vi "PicoLogDriver.vi"(1 "stop":bool) -> ()   [LabVIEW 2016]
uses:
  <vilib>/Platform/TimedLoop/XDataNode/timing_clust.ctl
  <vilib>/Platform/TimedLoop/XDataNode/nitl_modes.ctl
  <vilib>/Platform/TimedLoop/XDataNode/wakeup.ctl
  <vilib>/Utility/NIReport.llb/image depth.ctl
  Instance           1 30Saved   pl1000StreamingExample .vi
  <vilib>/Utility/NIReport.llb/Append Report Text (str wrap).vi
  <vilib>/printing/OpenHTMLReport.llb/Open HTML Report in Browser (Refnum).vi
  <vilib>/platform/TimedLoop/XDataNode/XDataNode.xnode
  <vilib>/Utility/NIReport.llb/NI_report.lvclass
  pl1000.dll
  <vilib>/Platform/TimedLoop/XDataNode/XDNodeRunTimeDep.lvlib
  <vilib>/Utility/NIReport.llb/NI_ReportGenerationCore.lvlib
panel:
  in  "Tab Control":enum32{"Real Time", "Over time"}(tab)
  out "Waveform Chart":dbl[][](graph)
  out "Vin":dbl format="%#.2f"
  out "Elapsed Time":string caption="Elapsed Time Text"
  out "Time variation Graph":waveform(dbl)[](graph)
  out "error out 2":errorcluster
  out "Boolean":bool
  out "Path":path
  in  "Period (microseconds)":u16=100 min=100 max=1800
  out "Triggered":bool
  out "No. of channels":i32
  in  "D3":bool=TRUE
  in  "D2":bool=TRUE
  in  "D1":bool=TRUE
  in  "D0":bool=TRUE
  in  "Enable auto trigger":bool
  in  "Trigger Enable":bool
  in  "Hysteresis (mV)":u32
  in  "Threshold (mV)":u32=1000
  in  "Trigger direction":u16(ring) items=["Rising", "Falling"]
  in  "Trigger channel":u16=1 min=1 max=16 step=1
  in  "Auto trigger time (ms)":u16=1000
  out "Sampling rate (S/s)":dbl
  in  "Channels Enabled (e.g 1,2,3,4) * use comma*":string="1,2,3,4,5"
  in  "Desired sample rate (S/s)":u32=100 max=100000
  # "Trigger Settings"
  # "CH5 - Vin"
  # "CH4 - temperature sensor"
  # "Current Values in mV"
  # "CH1"
  # "CH2"
  # "CH3"
  # "Temperature"
  # "@Vlad-Eusebiu Baciu"
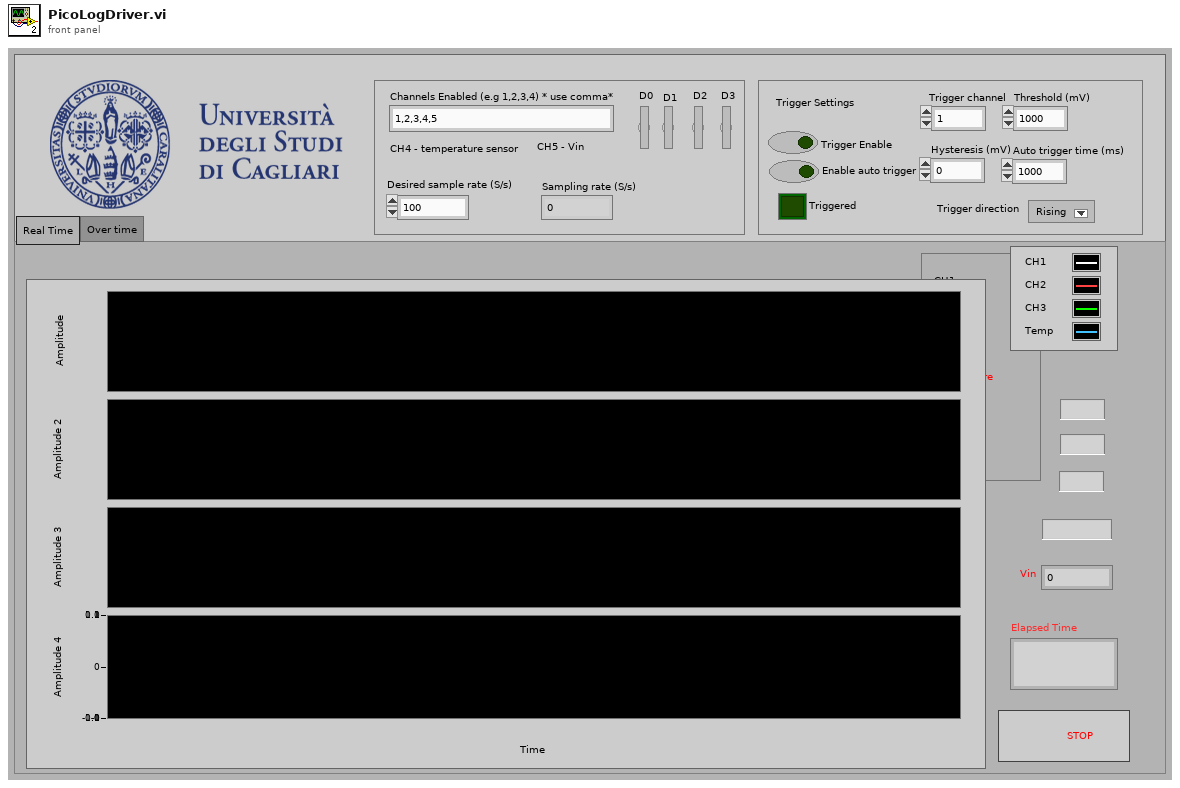
[diagram p1: front panel]
types:
  T1 = enum16{"open", "open or create", "create or replace", "create", "open (read-only)"}
  T2 = typedef "XDNodeRunTimeDep.lvlib/timing_clust.ctl" = cluster{"Expected End [f-1]":u64, "Actual End [f-1]":u64, "Finished Late? [f-1]":bool, "Expected End [i-1]":u64, "Actual End [i-1]":u64, "Finished Late? [i-1]":bool, "Expected Start [i]":u64, "Actual Start [i]":u64, "Expected Start [f]":u64, "Actual Start [f]":u64, "Source Name":string, "Structure Name":string, "Period":i64, "Deadline":i64, "Offset":i64, "Start":i64, "Priority":i32, "Timeout":i32, "Mode":T3, "Wakeup Reason":T4, "Error":errorcluster, "Source Type":string, "Secondary Source Type":string, "Global End Time":u64, "Global Start Time":u64, "Frame Duration":u64, "Iteration Duration":u64, "Assigned CPU":i32, "I/O Scan Engine Mode":u32}
  T3 = typedef "XDNodeRunTimeDep.lvlib/nitl_modes.ctl" = enum32{"No Change", "Process missed periods, maintain original phase", "Discard missed periods, maintain original phase", "Process missed periods, ignore original phase", "Discard missed periods, ignore original phase"}
  T4 = typedef "XDNodeRunTimeDep.lvlib/wakeup.ctl" = enum32{"Normal", "Aborted", "Asynchronous wakeup", "Timing source error", "Timed loop error", "Timeout"}
  T5 = enum8{"Enabled", "Disabled", "Disabled and Grayed Out"}
  T6 = enum16{"Standard Report", "HTML", "Word", "Excel"}
  T7 = typedef "NI_ReportGenerationCore.lvlib/image depth.ctl" = u16
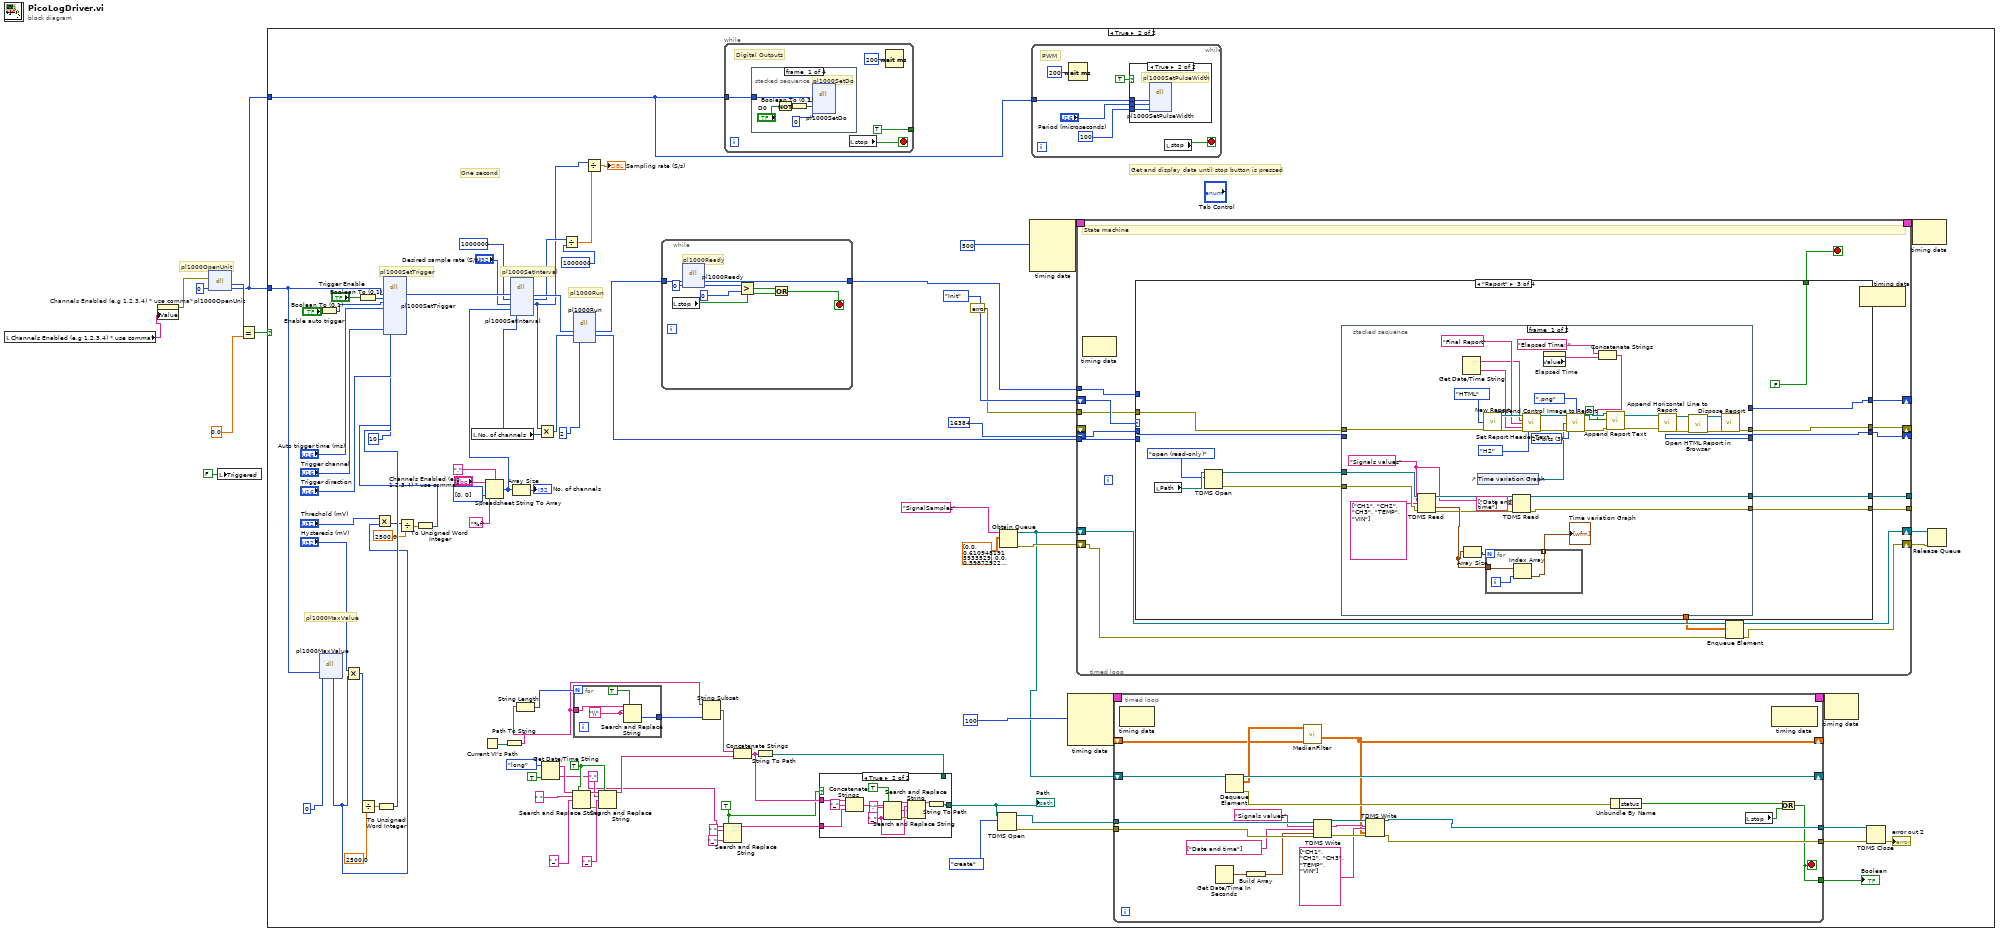
[diagram p0: block diagram]
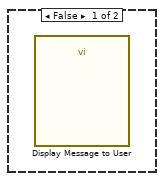
[diagram p2: hidden frame]
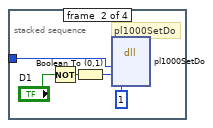
[diagram p5: hidden frame]
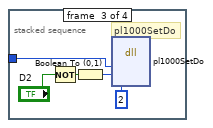
[diagram p6: hidden frame]
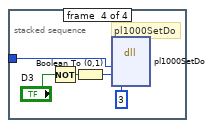
[diagram p7: hidden frame]
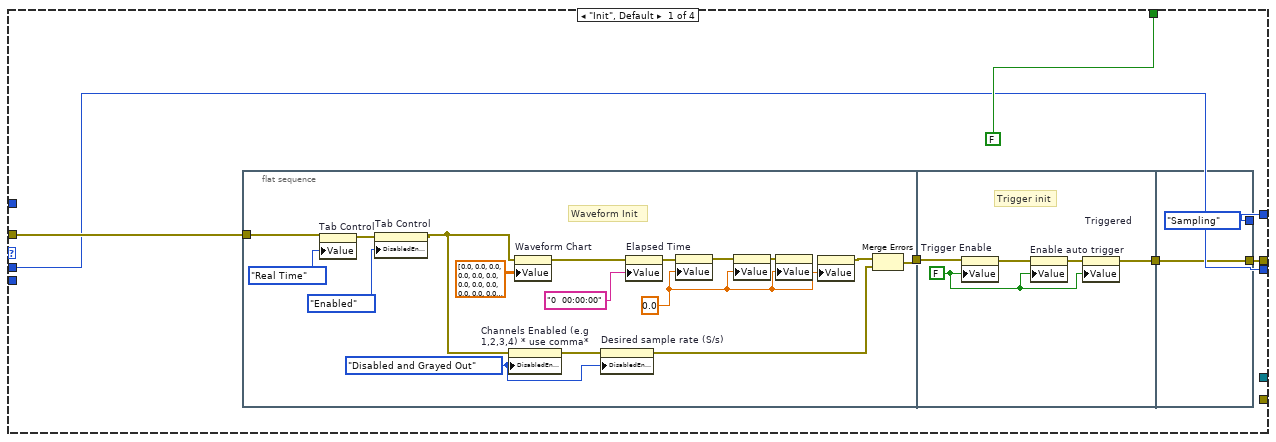
[diagram p8: hidden frame]
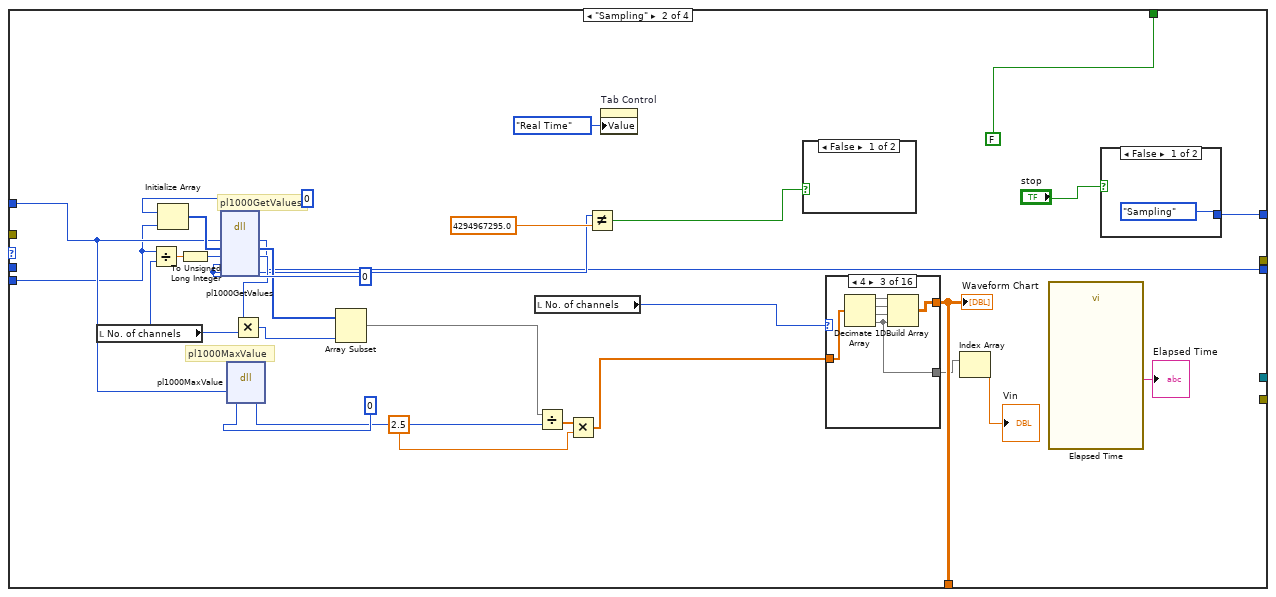
[diagram p9: hidden frame]
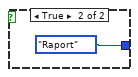
[diagram p10: hidden frame]
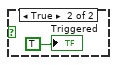
[diagram p11: hidden frame]
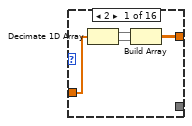
[diagram p12: hidden frame]
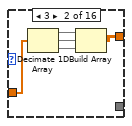
[diagram p13: hidden frame]
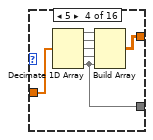
[diagram p14: hidden frame]
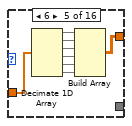
[diagram p15: hidden frame]
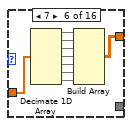
[diagram p16: hidden frame]
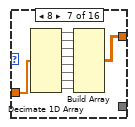
[diagram p17: hidden frame]
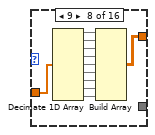
[diagram p18: hidden frame]
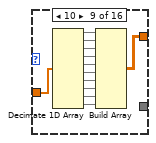
[diagram p19: hidden frame]
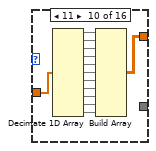
[diagram p20: hidden frame]
diagram:
  # "pl1000OpenUnit"
  n1 = local read "Channels Enabled (e.g 1,2,3,4) * use comma*"() -> (w1:string)
  n2 = property on="Channels Enabled (e.g 1,2,3,4) * use comma*" class="Str"("Value"=w1) -> (error out=w2:errorcluster)  [unwired: 2 in, 1 out]
  n3 = dll-call lib="E:/Erasmus practica/pl1000.dll" fn="pl1000OpenUnit"(error in=w2, "handle"=i16 0) -> ("status"=w5:u32, "handle"=w4:i16)  [unwired: 2 in, 2 out]
  n4 = local write "Triggered"(FALSE ("Boolean")) -> ()
  n5 = Equal?(x=w5, y=0.0) -> (x = y?=w7:bool)
  n6 = case shown="True" w7 {
    tunnel: w4 -> [_ w77]
    tunnel: w4 -> [_ w49]
    frame False {
      n7 = call "Display Message to User"() -> ()  [unwired: 10 in, 2 out]
    }
    frame True {
      w13 = TRUE ("replace all? (F)")
      w31 = TRUE ("replace all? (F)")
      # "Get and display data until stop button is pressed"
      # "One second"
      # "pl1000MaxValue"
      # "pl1000SetTrigger"
      # "pl1000Run"
      # "pl1000SetInterval"
      n8 = dll-call lib="E:/Erasmus practica/pl1000.dll" fn="pl1000MaxValue"("handle"=w77, "maxValue"=u16 0) -> ("maxValue"=w67:u16)  [unwired: 5 in, 2 out]
      n9 = Boolean To (0,1)(Boolean="Enable auto trigger") -> (0, 1=w57:i16)
      n10 = Multiply(x="Hysteresis (mV)", y=w67) -> (x*y=w79:u32)
      n11 = Boolean To (0,1)(Boolean="Trigger Enable") -> (0, 1=w65:i16)
      n12 = Divide(x=w79, y=2500.0) -> (x/y=w74:dbl)
      n13 = Multiply(x="Threshold (mV)", y=w67) -> (x*y=w70:u32)
      n14 = To Unsigned Word Integer(number=w74) -> (unsigned 16bit integer=w75:u16)
      n15 = Divide(x=w70, y=2500.0) -> (x/y=w71:dbl)
      n16 = To Unsigned Word Integer(number=w71) -> (unsigned 16bit integer=w68:u16)
      n17 = dll-call lib="E:/Erasmus practica/pl1000.dll" fn="pl1000SetTrigger"("handle"=w77, "enabled"=w65, "auto_trigger"=w57, "auto_ms"="Auto trigger time (ms)", "channel"="Trigger channel", "dir"="Trigger direction", "threshold"=w68, "hysteresis"=w75, "delay"=u16 10) -> ("handle"=w97:i16)  [unwired: 12 in, 2 out]
      n18 = local read "No. of channels"() -> (w62:i32)
      n19 = Current VI's Path() -> (path=w39:path)
      n20 = Spreadsheet String To Array(delimiter (Tab)=",", format string="%f", spreadsheet string="Channels Enabled (e.g 1,2,3,4) * use comma*", array type (2D Dbl)=u32[] [0, 0]) -> (array=w89:u32[])
      n21 = Path To String(path=w39) -> (string=w28:string)
      n22 = dll-call lib="E:/Erasmus practica/pl1000.dll" fn="pl1000SetInterval"("handle"=w97, "us_for_block"=u32 1000000, "ideal_no_of_samples"="Desired sample rate (S/s)", "channels"=w89, "no_of_channels"=w62) -> ("handle"=w94:i16, "us_for_block"=w84:u32, "ideal_no_of_samples"=w61:u32)  [unwired: 6 in, 2 out]
      n23 = Array Size(array=w89) -> (size(s)=→"No. of channels":i32)
      n24 = String Length(string=w28) -> (length=w30:i32)
      n25 = Multiply(x=w61, y=w62) -> (x*y=w60:u32)
      n26 = Get Date/Time String(date format (0)=enum16{"short", "long", "abbreviated"}."long", want seconds? (F)=TRUE) -> (date string=w37:string, time string=w23:string)  [unwired: 1 in]
      n27 = Divide(x=w84, y=u32 1000000) -> (x/y=w83:dbl)
      n28 = Search and Replace String(replace all?=w31, input string=w37, search string=" ", replace string="_" ("replace string (\"\")")) -> (result string=w35:string, error out=w25:errorcluster)  [unwired: 4 in, 2 out]
      n29 = dll-call lib="E:/Erasmus practica/pl1000.dll" fn="pl1000Run"("handle"=w94, "no_of_values"=w60, "method"=2) -> ("handle"=w95:i16, "no_of_values"=w86:u32)  [unwired: 5 in, 2 out]
      n30 = for {
        N: w30 -> [_]
        tunnel: w28 -> [w113]
        tunnel: [w112] -> w29
        w110 = "\\" ("regular expression")
        n31 = Search and Replace String(replace all?=TRUE ("replace all? (F)"), input string=w113, search string=w110, replace string=w110) -> (offset past replacement=w112:i32)  [unwired: 4 in, 3 out]
      }
      n32 = Divide(x=w61, y=w83) -> (x/y=→"Sampling rate (S/s)":dbl)
      n33 = Search and Replace String(replace all?=w31, input string=w35, search string=",", replace string="_" ("replace string (\"\")"), error in=w25) -> (result string=w27:string)  [unwired: 3 in, 3 out]
      n34 = while {
        tunnel: w95 -> [w512]
        tunnel: [w511] -> w93
        stop <- w507 stop-if-true
        # "pl1000Ready"
        n35 = local read "stop"() -> (w506:bool)
        n36 = dll-call lib="E:/Erasmus practica/pl1000.dll" fn="pl1000Ready"("handle"=w512, "ready"=i16 0) -> ("handle"=w511:i16, "ready"=w508:i16)  [unwired: 4 in, 2 out]
        n37 = Greater?(x=w508, y=i16 0) -> (0:w509:bool)
        n38 = Or(x=w509, y=w506) -> (x .or. y?=w507:bool)
      }
      n39 = String Subset(string=w28, length (rest)=w29) -> (substring=w26:string)  [unwired: 1 in]
      n40 = Search and Replace String(replace all?=w13, input string=w23, search string=" ", replace string="_" ("replace string (\"\")")) -> (result string=w20:string)  [unwired: 4 in, 3 out]
      n41 = while {
        tunnel: [TRUE] -> _
        tunnel: w49 -> [w150]
        stop <- w153 stop-if-true
        # "Digital Outputs"
        n42 = stacked-sequence {
          tunnel: w150 -> [w154 w159 w164 w169]
          frame #0 {
            # "pl1000SetDo"
            n43 = Not(x="D0") -> (.not. x?=w155:bool)
            n44 = Boolean To (0,1)(Boolean=w155) -> (0, 1=w157:i16)
            n45 = dll-call lib="E:/Erasmus practica/pl1000.dll" fn="pl1000SetDo"("handle"=w154, "do_value"=w157, "doNo"=i16 0) -> ()  [unwired: 7 in, 2 out]
          }
          frame #1 {
            # "pl1000SetDo"
            n46 = Not(x="D1") -> (.not. x?=w160:bool)
            n47 = Boolean To (0,1)(Boolean=w160) -> (0, 1=w162:i16)
            n48 = dll-call lib="E:/Erasmus practica/pl1000.dll" fn="pl1000SetDo"("handle"=w159, "do_value"=w162, "doNo"=i16 1) -> ()  [unwired: 7 in, 2 out]
          }
          frame #2 {
            # "pl1000SetDo"
            n49 = Not(x="D2") -> (.not. x?=w165:bool)
            n50 = Boolean To (0,1)(Boolean=w165) -> (0, 1=w167:i16)
            n51 = dll-call lib="E:/Erasmus practica/pl1000.dll" fn="pl1000SetDo"("handle"=w164, "do_value"=w167, "doNo"=i16 2) -> ()  [unwired: 7 in, 2 out]
          }
          frame #3 {
            # "pl1000SetDo"
            n52 = Not(x="D3") -> (.not. x?=w170:bool)
            n53 = Boolean To (0,1)(Boolean=w170) -> (0, 1=w172:i16)
            n54 = dll-call lib="E:/Erasmus practica/pl1000.dll" fn="pl1000SetDo"("handle"=w169, "do_value"=w172, "doNo"=i16 3) -> ()  [unwired: 7 in, 2 out]
          }
        }
        n55 = local read "stop"() -> (w153:bool)
        n56 = Wait (ms)(milliseconds to wait=u32 200) -> ()  [unwired: 1 out]
      }
      n57 = Concatenate Strings(w26, w27) -> (w24:string)
      n58 = String To Path(string=w24) -> (path=w12:path)
      n59 = case shown="True" w13 {
        tunnel: w24 -> [_ w109]
        tunnel: w20 -> [_ w107]
        tunnel: [w98 w106] -> w14
        tunnel: w12 -> [w98 _]
        frame False {
        }
        frame True {
          w101 = "_" ("replace string (\"\")")
          w100 = ":" ("search string")
          n60 = Concatenate Strings(w109, "_" ("string"), w107) -> (w105:string)
          n61 = Search and Replace String(replace all?=TRUE ("replace all? (F)"), input string=w105, search string=w100, replace string=w101) -> (result string=w102:string, error out=w103:errorcluster)  [unwired: 4 in, 2 out]
          n62 = Search and Replace String(input string=w102, search string=w101, replace string=w100, error in=w103) -> (result string=w99:string)  [unwired: 4 in, 3 out]
          n63 = String To Path(string=w99) -> (path=w106:path)
        }
      }
      "Path" <- w14
      n64 = TDMS Open(10:T1."create" ("operation (0:open)"), 11:w14) -> (0:w16:errorcluster, 3:w17:refnum<k34>)  [unwired: 5 in]
      n65 = Obtain Queue(name (unnamed)="SignalSamples", element data type=dbl[][] [[0.0, 0.6109481915933529, 0.0, 0.5987292277614858, 0.0, 0.6036168132942327, 0.0, 0.6085043988269795, 0.0, 0.6085043988269795, 0.0, 0.6133919843597263, 0.0, 0.6207233626588465, 0.0, 0.4056695992179863, 0.0, 0.4032258064516129, 0.0, 0.4032258064516129, 0.0, 0.4105571847507331, 0.0, 0.4105571847507331, 0.0, 0.4130009775171065, 0.0, 0.4130009775171065, 0.0, 0.760019550342131, 0.0, 0.8113391984359726, 0.0, 0.8015640273704789, 0.0, 0.8284457478005864, 0.0, 0.8357771260997067, 0.0, 0.8235581622678396, 0.0, 0.8553274682306939, 0.0, 0.8553274682306939, 0.0, 0.8651026392961878, 0.0, 0.8699902248289346, 0.0, 0.8846529814271751, 0.0, 0.8797653958944283, 0.0, 0.8822091886608017, 0.0, 0.8968719452590421, 0.0, 0.9090909090909092, 0.0, 0.8822091886608017, 0.0, 0.8870967741935485, 0.0, 0.8870967741935485, 0.0, 0.8822091886608017, 0.0, 0.9017595307917889, 0.0, 0.9188660801564028, 0.0, 0.9188660801564028, 0.0, 0.8944281524926687, 0.0, 0.926197458455523, 0.0, 0.9310850439882699, 0.0, 0.9726295210166178, 0.0, 0.9530791788856305, 0.0, 0.9506353861192571, 0.0, 0.9530791788856305, 0.0, 0.955522971652004, 0.0, 0.9848484848484849, 0.0, 0.9408602150537635, 0.0, 0.9530791788856305, 0.0, 0.9628543499511242, 0.0, 0.9530791788856305, 0.0, 0.967741935483871], [0.0, 0.0, 0.0, 0.0, 0.0, 0.0, 0.0, 0.0, 0.0, 0.0, 0.0, 0.0, 0.0, 0.0, 0.0, 0.0, 0.0, 0.0, 0.0, 0.0, 0.0, 0.0, 0.0, 0.0, 0.0, 0.0, 0.0, 0.0, 0.0, 0.0, 0.0, 0.0, 0.0, 0.0, 0.0, 0.0, 0.0, 0.0, 0.0, 0.0, 0.0, 0.0, 0.0, 0.0, 0.0, 0.0, 0.0, 0.0, 0.0, 0.0, 0.0, 0.0, 0.0, 0.0, 0.0, 0.0, 0.0, 0.0, 0.0, 0.0, 0.0, 0.0, 0.0, 0.0, 0.0, 0.0, 0.0, 0.0, 0.0, 0.0, 0.0, 0.0, 0.0, 0.0, 0.0, 0.0, 0.0, 0.0, 0.0, 0.0, 0.0, 0.0, 0.0, 0.0, 0.0, 0.0, 0.0, 0.0, 0.0, 0.0, 0.0, 0.0, 0.0, 0.0, 0.0, 0.0, 0.0, 0.0, 0.0, 0.0], [0.0, 0.0, 0.0, 0.0, 0.0, 0.0, 0.0, 0.0, 0.0, 0.0, 0.0, 0.0, 0.0, 0.0, 0.0, 0.0, 0.0, 0.0, 0.0, 0.0, 0.0, 0.0, 0.0, 0.0, 0.0, 0.0, 0.0, 0.0, 0.0, 0.0, 0.0, 0.0, 0.0, 0.0, 0.0, 0.0, 0.0, 0.0, 0.0, 0.0, 0.0, 0.0, 0.0, 0.0, 0.0, 0.0, 0.0, 0.0, 0.0, 0.0, 0.0, 0.0, 0.0, 0.0, 0.0, 0.0, 0.0, 0.0, 0.0, 0.0, 0.0, 0.0, 0.0, 0.0, 0.0, 0.0, 0.0, 0.0, 0.0, 0.0, 0.0, 0.0, 0.0, 0.0, 0.0, 0.0, 0.0, 0.0, 0.0, 0.0, 0.0, 0.0, 0.0, 0.0, 0.0, 0.0, 0.0, 0.0, 0.0, 0.0, 0.0, 0.0, 0.0, 0.0, 0.0, 0.0, 0.0, 0.0, 0.0, 0.0], [2.228739002932551, 2.228739002932551, 2.2311827956989245, 2.228739002932551, 2.2311827956989245, 2.228739002932551, 2.228739002932551, 2.228739002932551, 2.2311827956989245, 2.228739002932551, 2.228739002932551, 2.228739002932551, 2.228739002932551, 2.228739002932551, 2.228739002932551, 2.228739002932551, 2.228739002932551, 2.228739002932551, 2.228739002932551, 2.228739002932551, 2.228739002932551, 2.228739002932551, 2.228739002932551, 2.228739002932551, 2.228739002932551, 2.228739002932551, 2.228739002932551, 2.228739002932551, 2.228739002932551, 2.228739002932551, 2.228739002932551, 2.228739002932551, 2.228739002932551, 2.228739002932551, 2.228739002932551, 2.228739002932551, 2.228739002932551, 2.228739002932551, 2.228739002932551, 2.2262952101661777, 2.228739002932551, 2.2262952101661777, 2.228739002932551, 2.228739002932551, 2.228739002932551, 2.228739002932551, 2.228739002932551, 2.228739002932551, 2.228739002932551, 2.228739002932551, 2.228739002932551, 2.228739002932551, 2.228739002932551, 2.228739002932551, 2.228739002932551, 2.228739002932551, 2.228739002932551, 2.228739002932551, 2.228739002932551, 2.228739002932551, 2.228739002932551, 2.228739002932551, 2.228739002932551, 2.228739002932551, 2.228739002932551, 2.228739002932551, 2.228739002932551, 2.228739002932551, 2.228739002932551, 2.228739002932551, 2.228739002932551, 2.228739002932551, 2.228739002932551, 2.2262952101661777, 2.228739002932551, 2.228739002932551, 2.228739002932551, 2.228739002932551, 2.228739002932551, 2.228739002932551, 2.228739002932551, 2.228739002932551, 2.228739002932551, 2.228739002932551, 2.228739002932551, 2.228739002932551, 2.228739002932551, 2.228739002932551, 2.228739002932551, 2.228739002932551, 2.228739002932551, 2.228739002932551, 2.228739002932551, 2.228739002932551, 2.228739002932551, 2.228739002932551, 2.228739002932551, 2.228739002932551, 2.228739002932551, 2.228739002932551]] ("Waveform Chart")) -> (queue out=w41:refnum<queue>, error out=w42:errorcluster)  [unwired: 3 in, 1 out]
      n66 = node-c288(i64 500 ("Period")) -> (w55:T2)  [unwired: 3 in]
      n67 = while {
        tunnel: w49 -> [w146]
        stop <- w145 stop-if-true
        # "PWM"
        n68 = Wait (ms)(milliseconds to wait=u32 200) -> ()  [unwired: 1 out]
        n69 = case shown="True" TRUE {
          tunnel: w146 -> [_ w149]
          tunnel: "Period (microseconds)" -> [_ w148]
          tunnel: u8 100 ("Duty Cycle (%)") -> [_ w147]
          frame False {
          }
          frame True {
            # "pl1000SetPulseWidth"
            n70 = dll-call lib="E:/Erasmus practica/pl1000.dll" fn="pl1000SetPulseWidth"("handle"=w149, "period"=w148, "cycle"=w147) -> ()  [unwired: 7 in, 2 out]
          }
        }
        n71 = local read "stop"() -> (w145:bool)
      }
      n72 = node-c288(i64 100 ("Period")) -> (w48:T2)  [unwired: 3 in]
      n73 = timed-loop {
        tunnel: w86 -> [w188]
        tunnel: w93 -> [w189]
        timing: w55 -> [_]
        timing-out: [_] -> w54
        tunnel: errorcluster {"status"=FALSE, "code"=0, "source"=""} ("error constant") -> [w186]
        shift-right: [w185] -> _
        shift-left: _ -> [_]
        shift-right: [w184] -> _
        shift-left: enum16{"Init", "Sampling", "Raport", "Stop"}."Init" -> [w187]
        shift-right: [w183] -> _
        shift-left: i16 16384 ("handle") -> [w182]
        shift-right: [w179] -> w44
        shift-left: w41 -> [w180]
        shift-right: [w177] -> w43
        shift-left: w42 -> [w176]
        tunnel: [w175] -> _
        tunnel: [w174] -> _
        stop <- w181 stop-if-true
        # "State machine"
        n74 = node-c288() -> ()  [unwired: 1 in, 1 out]
        n75 = case shown="\"Raport\"" w187 {
          tunnel: w189 -> [_ w245 _ _]
          tunnel: w188 -> [_ w236 _ _]
          tunnel: w186 -> [w196 _ w428 w484]
          tunnel: [w194 _ w433 w478] -> w185
          tunnel: [w192 w228 w429 w477] -> w184
          tunnel: [w190 w226 w431 w481] -> w183
          tunnel: w182 -> [w190 _ w432 w485]
          tunnel: [FALSE ("stop") FALSE ("stop") FALSE ("stop") w482] -> w181
          tunnel: [_ w224 _ _] -> w178
          tunnel: [_ _ w427 _] -> w175
          tunnel: [_ _ w426 _] -> w174
          frame "Init", Default {
            n76 = flat-sequence {
              tunnel: w196 -> [w199]
              tunnel: [w202] -> w195
              tunnel: w195 -> [w218]
              tunnel: [w215] -> w193
              tunnel: [w220] -> w194
              tunnel: w193 -> [w220]
              tunnel: [enum16{"Init", "Sampling", "Raport", "Stop"}."Sampling"] -> w192
              frame #0 {
                w205 = T5."Disabled and Grayed Out" ("Disabled")
                w207 = 0.0 ("Value")
                # "Waveform Init"
                n77 = property on="Tab Control" class="TabCtl (strict)"(error in=w199, "Value"=enum32{"Real Time", "Over time"}."Real Time" ("Tab Control")) -> (error out=w198:errorcluster)  [unwired: 1 in, 1 out]
                n78 = property on="Tab Control" class="TabCtl (strict)"(error in=w198, "DisabledEnum"=T5."Enabled" ("Disabled")) -> (error out=w201:errorcluster)  [unwired: 1 in, 1 out]
                n79 = property on="Channels Enabled (e.g 1,2,3,4) * use comma*" class="Str"(error in=w201, "DisabledEnum"=w205) -> (error out=w206:errorcluster)  [unwired: 1 in, 1 out]
                n80 = property on="Waveform Chart" class="WFChart (strict)"(error in=w201, "Value"=dbl[][] [[0.0, 0.0, 0.0, 0.0, 0.0, 0.0, 0.0, 0.0, 0.0, 0.0, 0.0, 0.0, 0.0, 0.0, 0.0, 0.0, 0.0, 0.0, 0.0, 0.0, 0.0, 0.0, 0.0, 0.0, 0.0, 0.0, 0.0, 0.0, 0.0, 0.0, 0.0, 0.0, 0.0, 0.0, 0.0, 0.0, 0.0, 0.0, 0.0, 0.0, 0.0, 0.0, 0.0, 0.0, 0.0, 0.0, 0.0, 0.0, 0.0, 0.0, 0.0, 0.0, 0.0, 0.0, 0.0, 0.0, 0.0, 0.0, 0.0, 0.0, 0.0, 0.0, 0.0, 0.0, 0.0, 0.0, 0.0, 0.0, 0.0, 0.0, 0.0, 0.0, 0.0, 0.0, 0.0, 0.0, 0.0, 0.0, 0.0, 0.0, 0.0, 0.0, 0.0, 0.0, 0.0, 0.0, 0.0, 0.0, 0.0, 0.0, 0.0, 0.0, 0.0, 0.0, 0.0, 0.0, 0.0, 0.0, 0.0, 0.0], [0.0, 0.0, 0.0, 0.0, 0.0, 0.0, 0.0, 0.0, 0.0, 0.0, 0.0, 0.0, 0.0, 0.0, 0.0, 0.0, 0.0, 0.0, 0.0, 0.0, 0.0, 0.0, 0.0, 0.0, 0.0, 0.0, 0.0, 0.0, 0.0, 0.0, 0.0, 0.0, 0.0, 0.0, 0.0, 0.0, 0.0, 0.0, 0.0, 0.0, 0.0, 0.0, 0.0, 0.0, 0.0, 0.0, 0.0, 0.0, 0.0, 0.0, 0.0, 0.0, 0.0, 0.0, 0.0, 0.0, 0.0, 0.0, 0.0, 0.0, 0.0, 0.0, 0.0, 0.0, 0.0, 0.0, 0.0, 0.0, 0.0, 0.0, 0.0, 0.0, 0.0, 0.0, 0.0, 0.0, 0.0, 0.0, 0.0, 0.0, 0.0, 0.0, 0.0, 0.0, 0.0, 0.0, 0.0, 0.0, 0.0, 0.0, 0.0, 0.0, 0.0, 0.0, 0.0, 0.0, 0.0, 0.0, 0.0, 0.0], [0.0024437927663734115, 0.0, 0.0024437927663734115, 0.0, 0.0024437927663734115, 0.0, 0.0024437927663734115, 0.0, 0.0024437927663734115, 0.0, 0.0024437927663734115, 0.0, 0.0024437927663734115, 0.0, 0.0024437927663734115, 0.0, 0.0024437927663734115, 0.0, 0.0024437927663734115, 0.0, 0.0024437927663734115, 0.0, 0.0024437927663734115, 0.0, 0.0024437927663734115, 0.0, 0.0024437927663734115, 0.0, 0.0024437927663734115, 0.0, 0.0024437927663734115, 0.0, 0.0024437927663734115, 0.0, 0.0024437927663734115, 0.0, 0.0024437927663734115, 0.0, 0.0024437927663734115, 0.0, 0.0024437927663734115, 0.0, 0.0024437927663734115, 0.0, 0.0024437927663734115, 0.0, 0.0024437927663734115, 0.0, 0.0024437927663734115, 0.0, 0.0024437927663734115, 0.0, 0.0024437927663734115, 0.0, 0.0024437927663734115, 0.0, 0.0024437927663734115, 0.0, 0.0024437927663734115, 0.0, 0.0024437927663734115, 0.0, 0.0024437927663734115, 0.0, 0.0024437927663734115, 0.0, 0.0024437927663734115, 0.0, 0.0024437927663734115, 0.0, 0.0024437927663734115, 0.0, 0.0024437927663734115, 0.0, 0.0024437927663734115, 0.0, 0.0024437927663734115, 0.0, 0.0024437927663734115, 0.0, 0.0024437927663734115, 0.0, 0.0024437927663734115, 0.0, 0.0024437927663734115, 0.0, 0.0024437927663734115, 0.0, 0.0024437927663734115, 0.0, 0.0024437927663734115, 0.0, 0.0024437927663734115, 0.0, 0.0024437927663734115, 0.0, 0.0024437927663734115, 0.0, 0.0024437927663734115, 0.0]] ("Waveform Chart")) -> (error out=w211:errorcluster)  [unwired: 1 in, 1 out]
                n81 = property on="Desired sample rate (S/s)" class="DigNum (strict)"(error in=w206, "DisabledEnum"=w205) -> (error out=w203:errorcluster)  [unwired: 1 in, 1 out]
                n82 = property on="Elapsed Time" class="Str"(error in=w211, "Value"="0  00:00:00" ("Elapsed Time Text")) -> (error out=w210:errorcluster)  [unwired: 1 in, 1 out]
                n83 = property class="DigNum (strict)"(error in=w210, "Value"=w207) -> (error out=w209:errorcluster)  [unwired: 1 in, 1 out]
                n84 = property class="DigNum (strict)"(error in=w209, "Value"=w207) -> (error out=w208:errorcluster)  [unwired: 1 in, 1 out]
                n85 = property class="DigNum (strict)"(error in=w208, "Value"=w207) -> ()  [unwired: 1 in, 2 out]
                n86 = property class="DigNum (strict)"("Value"=w207) -> (error out=w204:errorcluster)  [unwired: 2 in, 1 out]
                n87 = Merge Errors(w204, w203) -> (w202:errorcluster)
              }
              frame #1 {
                w214 = FALSE ("Trigger Enable")
                # "Trigger init"
                n88 = property on="Trigger Enable" class="Bool (strict)"(error in=w218, "Value"=w214) -> (error out=w217:errorcluster)  [unwired: 1 in, 1 out]
                n89 = property on="Enable auto trigger" class="Bool (strict)"(error in=w217, "Value"=w214) -> (error out=w216:errorcluster)  [unwired: 1 in, 1 out]
                n90 = property on="Triggered" class="Bool (strict)"(error in=w216, "Value"=w214) -> (error out=w215:errorcluster)  [unwired: 1 in, 1 out]
              }
              frame #2 {
              }
            }
          }
          frame "Sampling" {
            w250 = u16 0 ("values")
            # "pl1000MaxValue"
            # "pl1000GetValues"
            n91 = local read "No. of channels"() -> (w235:i32)
            n92 = Divide(x=w236, y=w235) -> (x/y=w238:dbl)
            n93 = Initialize Array(u16 0 ("element"), w236) -> (w249:u16[])
            n94 = To Unsigned Long Integer(number=w238) -> (unsigned 32bit integer=w237:u32)
            n95 = dll-call lib="E:/Erasmus practica/pl1000.dll" fn="pl1000GetValues"("handle"=w245, "values"=w249, "noOfValues"=w237, "overflow"=w250, "triggerIndex"=w250) -> ("handle"=w226:i16, "values"=w246:u16[], "noOfValues"=w234:u32, "triggerIndex"=w230:u32)  [unwired: 5 in, 2 out]
            n96 = dll-call lib="E:/Erasmus practica/pl1000.dll" fn="pl1000MaxValue"("handle"=w245, "maxValue"=u16 0) -> ("maxValue"=w243:u16)  [unwired: 5 in, 2 out]
            n97 = Multiply(x=w234, y=w235) -> (x*y=w233:u32)
            n98 = Array Subset(array=w246, length=w233) -> (w239:u16[])  [unwired: 1 in]
            n99 = local read "No. of channels"() -> (w247:i32)
            n100 = Divide(x=w239, y=w243) -> (x/y=w242:dbl[])
            n101 = Multiply(x=w242, y=2.5) -> (x*y=w240:dbl[])
            n102 = Not Equal?(x=w230, y=4294967295.0) -> (x != y?=w232:bool)
            n103 = property on="Tab Control" class="TabCtl (strict)"("Value"=enum32{"Real Time", "Over time"}."Real Time" ("Tab Control")) -> ()  [unwired: 2 in, 2 out]
            n104 = case shown="False" w232 {
              frame False {
              }
              frame True {
                "Triggered" <- TRUE ("Boolean")
              }
            }
            n105 = case shown="4" w247 {
              tunnel: [w255 w262 w266 w273 w281 w290 w300 w311 w323 w336 w350 w365 w381 w398 w416 w420] -> w224
              tunnel: w240 -> [w254 w261 w264 w270 w276 w284 w293 w303 w314 w326 w339 w353 w368 w384 w401 w419]
              tunnel: [_ _ w263 w269 _ _ _ _ _ _ _ _ _ _ _ _] -> w223
              frame 2 {
                n106 = Decimate 1D Array(w254) -> (w257:dbl[], w256:dbl[])
                n107 = Build Array(w257, w256) -> (w255:dbl[][])
              }
              frame 3 {
                n108 = Decimate 1D Array(w261) -> (w259:dbl[], w258:dbl[], w260:dbl[])
                n109 = Build Array(w259, w258, w260) -> (w262:dbl[][])
              }
              frame 4 {
                n110 = Decimate 1D Array(w264) -> (w268:dbl[], w267:dbl[], w265:dbl[], w263:dbl[])
                n111 = Build Array(w268, w267, w265, w263) -> (w266:dbl[][])
              }
              frame 5 {
                n112 = Decimate 1D Array(w270) -> (w275:dbl[], w274:dbl[], w272:dbl[], w271:dbl[], w269:dbl[])
                n113 = Build Array(w275, w274, w272, w271, w269) -> (w273:dbl[][])
              }
              frame 6 {
                n114 = Decimate 1D Array(w276) -> (w283:dbl[], w282:dbl[], w280:dbl[], w279:dbl[], w278:dbl[], w277:dbl[])
                n115 = Build Array(w283, w282, w280, w279, w278, w277) -> (w281:dbl[][])
              }
              frame 7 {
                n116 = Decimate 1D Array(w284) -> (w292:dbl[], w291:dbl[], w289:dbl[], w288:dbl[], w287:dbl[], w286:dbl[], w285:dbl[])
                n117 = Build Array(w292, w291, w289, w288, w287, w286, w285) -> (w290:dbl[][])
              }
              frame 8 {
                n118 = Decimate 1D Array(w293) -> (w302:dbl[], w301:dbl[], w299:dbl[], w298:dbl[], w297:dbl[], w296:dbl[], w295:dbl[], w294:dbl[])
                n119 = Build Array(w302, w301, w299, w298, w297, w296, w295, w294) -> (w300:dbl[][])
              }
              frame 9 {
                n120 = Decimate 1D Array(w303) -> (w313:dbl[], w312:dbl[], w310:dbl[], w309:dbl[], w308:dbl[], w307:dbl[], w306:dbl[], w305:dbl[], w304:dbl[])
                n121 = Build Array(w313, w312, w310, w309, w308, w307, w306, w305, w304) -> (w311:dbl[][])
              }
              frame 10 {
                n122 = Decimate 1D Array(w314) -> (w325:dbl[], w324:dbl[], w322:dbl[], w321:dbl[], w320:dbl[], w319:dbl[], w318:dbl[], w317:dbl[], w316:dbl[], w315:dbl[])
                n123 = Build Array(w325, w324, w322, w321, w320, w319, w318, w317, w316, w315) -> (w323:dbl[][])
              }
              frame 11 {
                n124 = Decimate 1D Array(w326) -> (w338:dbl[], w337:dbl[], w335:dbl[], w334:dbl[], w333:dbl[], w332:dbl[], w331:dbl[], w330:dbl[], w329:dbl[], w328:dbl[], w327:dbl[])
                n125 = Build Array(w338, w337, w335, w334, w333, w332, w331, w330, w329, w328, w327) -> (w336:dbl[][])
              }
              frame 12 {
                n126 = Decimate 1D Array(w339) -> (w352:dbl[], w351:dbl[], w349:dbl[], w348:dbl[], w347:dbl[], w346:dbl[], w345:dbl[], w344:dbl[], w343:dbl[], w342:dbl[], w341:dbl[], w340:dbl[])
                n127 = Build Array(w352, w351, w349, w348, w347, w346, w345, w344, w343, w342, w341, w340) -> (w350:dbl[][])
              }
              frame 13 {
                n128 = Decimate 1D Array(w353) -> (w367:dbl[], w366:dbl[], w364:dbl[], w363:dbl[], w362:dbl[], w361:dbl[], w360:dbl[], w359:dbl[], w358:dbl[], w357:dbl[], w356:dbl[], w355:dbl[], w354:dbl[])
                n129 = Build Array(w367, w366, w364, w363, w362, w361, w360, w359, w358, w357, w356, w355, w354) -> (w365:dbl[][])
              }
              frame 14 {
                n130 = Decimate 1D Array(w368) -> (w383:dbl[], w382:dbl[], w380:dbl[], w379:dbl[], w378:dbl[], w377:dbl[], w376:dbl[], w375:dbl[], w374:dbl[], w373:dbl[], w372:dbl[], w371:dbl[], w370:dbl[], w369:dbl[])
                n131 = Build Array(w383, w382, w380, w379, w378, w377, w376, w375, w374, w373, w372, w371, w370, w369) -> (w381:dbl[][])
              }
              frame 15 {
                n132 = Decimate 1D Array(w384) -> (w400:dbl[], w399:dbl[], w397:dbl[], w396:dbl[], w395:dbl[], w394:dbl[], w393:dbl[], w392:dbl[], w391:dbl[], w390:dbl[], w389:dbl[], w388:dbl[], w387:dbl[], w386:dbl[], w385:dbl[])
                n133 = Build Array(w400, w399, w397, w396, w395, w394, w393, w392, w391, w390, w389, w388, w387, w386, w385) -> (w398:dbl[][])
              }
              frame 16 {
                n134 = Decimate 1D Array(w401) -> (w418:dbl[], w417:dbl[], w415:dbl[], w414:dbl[], w413:dbl[], w412:dbl[], w411:dbl[], w410:dbl[], w409:dbl[], w408:dbl[], w407:dbl[], w406:dbl[], w405:dbl[], w404:dbl[], w403:dbl[], w402:dbl[])
                n135 = Build Array(w418, w417, w415, w414, w413, w412, w411, w410, w409, w408, w407, w406, w405, w404, w403, w402) -> (w416:dbl[][])
              }
              frame 1, Default {
                n136 = Decimate 1D Array(w419) -> (w421:dbl[])
                n137 = Build Array(w421) -> (w420:dbl[][])
              }
            }
            "Waveform Chart" <- w224
            n138 = Index Array(array=w223) -> (element=→"Vin":dbl)  [unwired: 1 in]
            n139 = call "Elapsed Time"() -> ("Elapsed Time Text"=→"Elapsed Time":string)  [unwired: 12 in, 7 out]
            n140 = case shown="False" "stop" {
              tunnel: [enum16{"Init", "Sampling", "Raport", "Stop"}."Sampling" enum16{"Init", "Sampling", "Raport", "Stop"}."Raport"] -> w228
              frame False {
              }
              frame True {
              }
            }
          }
          frame "Raport" {
            n141 = local read "Path"() -> (w425:path)
            n142 = TDMS Open(10:T1."open (read-only)" ("operation (0:open)"), 11:w425) -> (0:w423:errorcluster, 3:w422:refnum<k34>)  [unwired: 5 in]
            n143 = stacked-sequence {
              tunnel: [w454 _] -> w433
              tunnel: w428 -> [w470 _]
              tunnel: [_ w476] -> w431
              tunnel: w432 -> [_ w476]
              tunnel: [_ enum16{"Init", "Sampling", "Raport", "Stop"}."Stop"] -> w429
              tunnel: [w438 _] -> w427
              tunnel: [w439 _] -> w426
              tunnel: w423 -> [w447 _]
              tunnel: w422 -> [w446 _]
              frame #0 {
                w436 = "Signals values" ("group name in (Untitled)")
                w464 = T7 3 items=["B&W", "4 bits", "8 bits", "24 bits"] ("image depth")
                n144 = TDMS Read(0:w446, 5:w436, 7:string[] ["CH1", "CH2", "CH3", "TEMP", "VIN"] ("channel name(s) in"), 11:w447) -> (4:w437:refnum<k34>, 10:w443:waveform(dbl)[], 15:w440:errorcluster)  [unwired: 4 in, 3 out]
                n145 = Get Date/Time String() -> (date string=w449:string, time string=w448:string)  [unwired: 3 in]
                n146 = Array Size(array=w443) -> (size(s)=w444:i32)
                n147 = control-ref of="Time variation Graph"() -> (w441:refnum<vi>)
                n148 = call <vilib>:"New Report.vi"("report type"=T6."HTML", "error in (no error)"=w470) -> ("report out"=w468:refnum<class "NI_report.lvclass">, "error out"=w469:errorcluster)  [unwired: 12 in]
                n149 = for {
                  N: w444 -> [_]
                  tunnel: w443 -> [w473]
                  tunnel: [w472] -> w442 mode=indexing
                  i -> [w474]
                  n150 = Index Array(array=w473, index=w474) -> (element=w472:waveform(dbl))
                }
                "Time variation Graph" <- w442
                n151 = TDMS Read(0:w437, 5:w436, 7:string[] ["Date and time"] ("channel name(s) in"), 11:w440) -> (4:w438:refnum<k34>, 15:w439:errorcluster)  [unwired: 4 in, 4 out]
                n152 = call-dynamic "Set Report Header Text.vi"("report in"=w468, "left header text"=w449, "center header text"="Final Report", "right header text"=w448, "error in (no error)"=w469, "HTML header size"=enum16{"H1", "H2", "H3", "H4", "H5", "H6", "H7"}."H2") -> ("report out"=w466:refnum<class "NI_report.lvclass">, "error out"=w465:errorcluster)  [unwired: 8 in]
                n153 = property on="Elapsed Time" class="Str"() -> ("Value"=w434:string)  [unwired: 2 in, 2 out]
                n154 = call-dynamic "Append Control Image to Report.vi"("report in"=w466, "image file type (.jpg)"=enum16{".jpg", ".png"}.".png", "image depth"=w464, "ctrl reference"=w441, "error in (no error)"=w465) -> ("report out"=w453:refnum<class "NI_report.lvclass">, "error out"=w461:errorcluster)  [unwired: 7 in, 2 out]
                n155 = Concatenate Strings("Elapsed Time: ", w434) -> (w451:string)
                n156 = call-poly <vilib>:"Append Report Text.vi"("report in"=w453, "text"=w451, "append on new line? (F)"=TRUE, "error in (no error)"=w461) -> ("report out"=w459:refnum<class "NI_report.lvclass">, "error out"=w460:errorcluster)  [unwired: 8 in, 2 out]
                n157 = call-dynamic "Append Horizontal Line to Report.vi"("report in"=w459, "error in (no error)"=w460) -> ("report out"=w458:refnum<class "NI_report.lvclass">, "error out"=w457:errorcluster)  [unwired: 12 in]
                n158 = call-poly <vilib>:"Open HTML Report in Browser.vi"("report in"=w458, "error in (no error)"=w457) -> ("report out"=w456:refnum<class "NI_report.lvclass">, "error out"=w455:errorcluster)  [unwired: 11 in, 1 out]
                n159 = call-dynamic "Dispose Report.vi"("report in"=w456, "error in (no error)"=w455) -> ("error out"=w454:errorcluster)  [unwired: 13 in]
              }
              frame #1 {
              }
            }
          }
          frame "Stop" {
            n160 = dll-call lib="E:/Erasmus practica/pl1000.dll" fn="pl1000Stop"(error in=w484, "handle"=w485) -> (error out=w483:errorcluster, "handle"=w486:i16)  [unwired: 3 in, 1 out]
            n161 = stacked-sequence {
              tunnel: w486 -> [w490 _]
              tunnel: w483 -> [w489 w498]
              tunnel: [w488 _] -> w479
              tunnel: [_ TRUE ("stop")] -> w482
              tunnel: [w487 _] -> w481
              tunnel: [_ w491] -> w480
              tunnel: [_ enum16{"Init", "Sampling", "Raport", "Stop"}."Raport"] -> w477
              frame #0 {
                # "pl1000CloseUnit"
                n162 = dll-call lib="E:/Erasmus practica/pl1000.dll" fn="pl1000CloseUnit"(error in=w489, "handle"=w490) -> (error out=w488:errorcluster, "handle"=w487:i16)  [unwired: 3 in, 1 out]
              }
              frame #1 {
                w496 = T5."Enabled" ("Disabled")
                n163 = local write "stop"(FALSE ("stop")) -> ()
                n164 = property on="Channels Enabled (e.g 1,2,3,4) * use comma*" class="Str"(error in=w498, "DisabledEnum"=w496) -> (error out=w497:errorcluster)  [unwired: 1 in, 1 out]
                n165 = property on="Desired sample rate (S/s)" class="DigNum (strict)"(error in=w497, "DisabledEnum"=w496) -> (error out=w492:errorcluster)  [unwired: 1 in, 1 out]
                n166 = property on="Tab Control" class="TabCtl (strict)"(error in=w492, "Value"=enum32{"Real Time", "Over time"}."Over time" ("Tab Control")) -> (error out=w491:errorcluster)  [unwired: 1 in, 1 out]
              }
            }
            n167 = Merge Errors(w480, w479) -> (w478:errorcluster)
          }
        }
        n168 = Enqueue Element(queue=w180, element=w178, error in (no error)=w176) -> (queue out=w179:refnum<queue>, error out=w177:errorcluster)  [unwired: 1 in, 1 out]
        n169 = node-c288() -> ()  [unwired: 1 in, 1 out]
      }
      n170 = timed-loop {
        timing: w48 -> [_]
        timing-out: [_] -> w47
        shift-right: [w133] -> _
        shift-left: w41 -> [w134]
        tunnel: w17 -> [w128]
        tunnel: w16 -> [w129]
        tunnel: [w122] -> w15
        tunnel: [w120] -> w11
        shift-right: [w116] -> _
        shift-left: _ -> [w115]
        tunnel: [w114] -> w10
        stop <- w114 stop-if-true
        n171 = node-c288() -> ()  [unwired: 1 in, 1 out]
        n172 = Get Date/Time In Seconds() -> (seconds since 1Jan1904=w126:timestamp)
        n173 = Dequeue Element(queue=w134) -> (queue out=w133:refnum<queue>, element=w117:dbl[][], error out=w132:errorcluster)  [unwired: 2 in, 1 out]
        n174 = Build Array(w126) -> (w125:timestamp[])
        n175 = call "MedianFilter.vi"("last array 2"=w115, "Waveform Chart"=w117) -> ("output array"=w116:dbl[][])  [unwired: 9 in]
        n176 = TDMS Write(0:w128, 5:"Signals values" ("group name in (Untitled)"), 7:string[] ["Date and time"] ("channel name(s) in (Untitled)"), 9:w125, 11:w129) -> (4:w123:refnum<k34>, 6:w119:string, 15:w124:errorcluster)  [unwired: 1 in, 1 out]
        n177 = TDMS Write(0:w123, 5:w119, 7:string[] ["CH1", "CH2", "CH3", "TEMP", "VIN"] ("channel name(s) in (Untitled)"), 9:w116, 11:w124) -> (4:w122:refnum<k34>, 15:w120:errorcluster)  [unwired: 1 in, 2 out]
        n178 = Unbundle By Name(w132) -> ("status"=w131:bool)
        n179 = local read "stop"() -> (w130:bool)
        n180 = node-c288() -> ()  [unwired: 1 in, 1 out]
        n181 = Or(x=w131, y=w130) -> (x .or. y?=w114:bool)
      }
      "Boolean" <- w10
      n182 = node-c288(w47) -> ()  [unwired: 1 out]
      n183 = TDMS Close(8:w11, 11:w15) -> (0:→"error out 2":errorcluster)  [unwired: 1 out]
      n184 = node-c288(w54) -> ()  [unwired: 1 out]
      n185 = Release Queue(queue=w44, error in (no error)=w43) -> ()  [unwired: 1 in, 3 out]
    }
  }
